vi "Get HP 53132 Data.vi"(7 "error in (no error)":errorcluster, 9 "Channels to measure":i32[](array[numeric])=[1], 10 "VISA Resource Name":refnum<visa-resource-name>) -> (0 "error out":errorcluster, 2 "Data":dbl format="%#_10g", 3 "VISA Resource Name Out":refnum<visa-resource-name>)   [LabVIEW 2021]
uses:
  GPIB/VISA  Send Receive.vi
  Simple VISA Reader/Simple VISA Reader Driver.lvclass
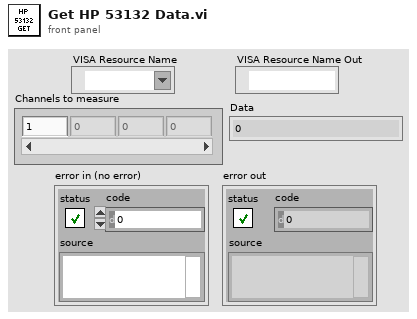
[diagram p1: front panel]
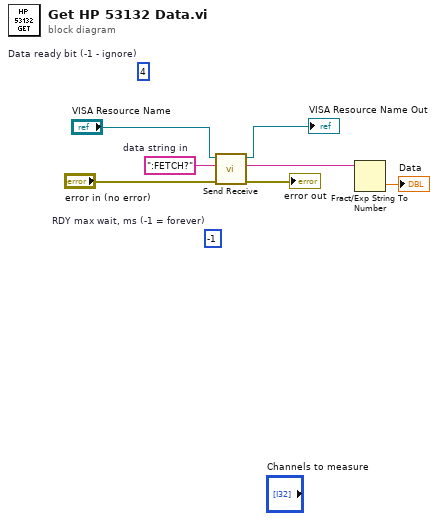
[diagram p0: block diagram]
diagram:
  (unwired) -1  # RDY max wait, ms (-1 = forever)
  (unwired) 4  # Data ready bit (-1 - ignore)
  w6 = ":FETCH?"  # data string in
  n1 = call-poly "Send Receive.vi"("error in (no error)"="error in (no error)", "data string in"=w6, "VISA Resource Name"="VISA Resource Name") -> ("error out"=→"error out":errorcluster, "data string out"=w4:string, "VISA Resource Name Out"=→"VISA Resource Name Out":refnum<visa-resource-name>)  [unwired: 6 in]
  n2 = Fract/Exp String To Number(string=w4) -> (number=→"Data":dbl)  [unwired: 4 out]
